vi "SetParam.vi"(8 "error in (no error)":errorcluster caption="entrée d'erreur (pas d'erreur)", 10 "Normalizer":cluster{"norm":string, "copy":bool}={"norm"="l2", "copy"=TRUE}, 11 "Normalizer.lvclass":refnum<class "Normalizer.lvclass">) -> (0 "error out":errorcluster caption="sortie d'erreur", 3 "Normalizer.lvclass":refnum<class "Normalizer.lvclass">)   [LabVIEW 2020, in "Normalizer.lvclass"]
doc: "Set Parameters"
uses:
  Normalizer.lvclass
  Normalizer.lvclass/Normalizer.ctl
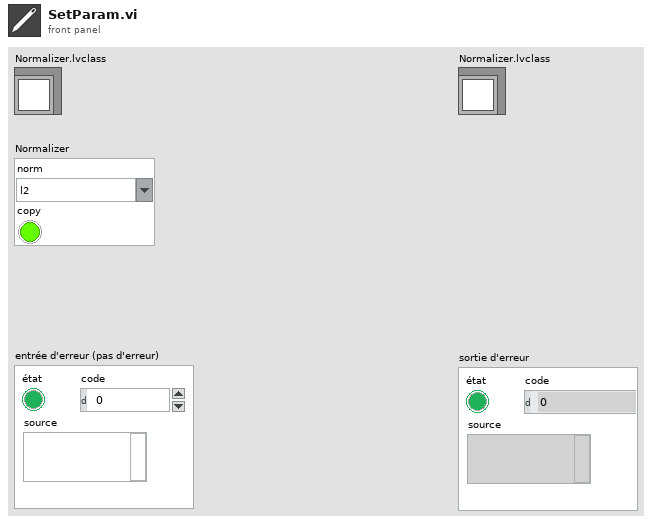
[diagram p1: front panel]
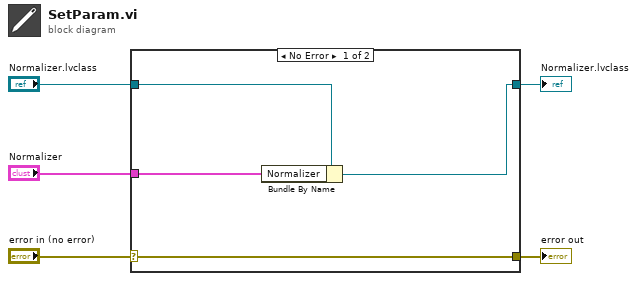
[diagram p0: block diagram]
diagram:
  n1 = case shown="No Error" "error in (no error)" {
    selector: "error in (no error)" -> [w9 w10]
    tunnel: [w9 w10] -> w4
    tunnel: [w7 w11] -> w2
    tunnel: "Normalizer.lvclass" -> [w8 w11]
    tunnel: "Normalizer" -> [w6 _]
    frame No Error {
      n2 = Bundle By Name(cluster=w8, "Normalizer"=w6) -> (w7:refnum<class "Normalizer.lvclass">)
    }
    frame Error {
    }
  }
  "error out" <- w4
  "Normalizer.lvclass" <- w2
